vi "BRig_dataLC_Reward_Delay_l1.vi"() -> (2 "output_Reward_Delay":i32)   [LabVIEW 2014]
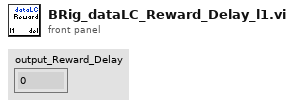
[diagram p1: front panel]
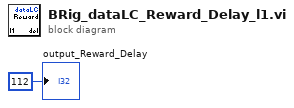
[diagram p0: block diagram]
diagram:
  "output_Reward_Delay" <- 112 ("output_iBlock")
